vi "CH_LM Reset.vi"(0 "Meter Index":i32, 2 "Password":string, 5 "error in (no error)":errorcluster, 7 "Timeout / ms (3000)":i32=3000, 9 "Lock Timeout / ms (1000)":i32=1000) -> (11 "Lock timed out":bool, 14 "Meter Index":i32, 19 "error out":errorcluster)   [LabVIEW 2012, in "CH_LM.lvlib"]
doc: "Resets the instrument and then sends a set of default setup commands to the instrument.\n\n<B>Hint:</B> Because this command will reset the realtime clock it is a password protected command that can be issued only after setting the calibration password."
uses:
  CH_LM.lvlib
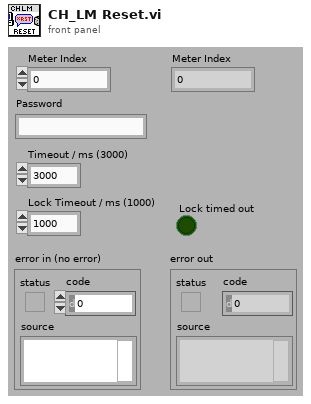
[diagram p1: front panel]
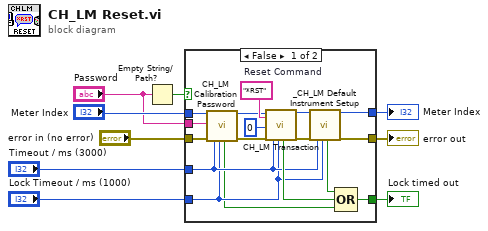
[diagram p0: block diagram]
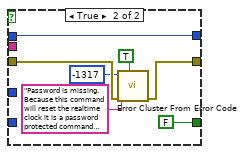
[diagram p2: hidden frame]
diagram:
  n1 = Empty String/Path?(string/path="Password") -> (empty?=w1:bool)
  n2 = case shown="False" w1 {
    tunnel: [w21 FALSE] -> w9
    tunnel: [w19 w33] -> w8
    tunnel: [w18 w30] -> w7
    tunnel: "Meter Index" -> [w17 w33]
    tunnel: "error in (no error)" -> [w15 w31]
    tunnel: "Timeout / ms (3000)" -> [w13 _]
    tunnel: "Lock Timeout / ms (1000)" -> [w12 _]
    tunnel: "Password" -> [w10 _]
    frame False {
      w24 = "*RST"  # Reset Command
      n3 = call "CH_LM Calibration Password.vi"("Meter Index"=w17, "Password"=w10, "error in (no error)"=w15, "Timeout / ms (3000)"=w13, "Lock Timeout / ms (1000)"=w12) -> ("Lock timed out"=w11:bool, "Meter Index"=w16:i32, "error out"=w14:errorcluster)  [unwired: 12 out]
      n4 = call "CH_LM Transaction.vi"("Meter Index"=w16, "Command String"=w24, "NofStrings (-1:all)"=0, "error in (no error)"=w14, "Timeout / ms (3000)"=w13, "Lock Timeout / ms (1000)"=w12) -> ("Lock timed out"=w22:bool, "Meter Index"=w25:i32, "error out"=w26:errorcluster)  [unwired: 11 out]
      n5 = call "_CH_LM Default Instrument Setup.vi"("Meter Index"=w25, "error in (no error)"=w26, "Timeout / ms (3000)"=w13, "Lock Timeout / ms (1000)"=w12) -> ("Lock timed out"=w23:bool, "Meter Index"=w19:i32, "error out"=w18:errorcluster)  [unwired: 13 out]
      n6 = Compound Arithmetic op=OR(w23, w22, w11) -> (w21:bool)
    }
    frame True {
      n7 = call <vilib>:"Error Cluster From Error Code.vi"("show call chain? (False)"=TRUE, "error in (no error)"=w31, "error message (\"\")"="Password is missing. Because this command will reset the realtime clock it is a password protected command that can be issued only after setting the calibration password." ("error message (\"\")"), "error code (0)"=-1317) -> ("error out"=w30:errorcluster)  [unwired: 5 out]
    }
  }
  "error out" <- w7
  "Meter Index" <- w8
  "Lock timed out" <- w9
